vi "GetAssetList.vi"(7 "LabVIEW Web Service Request":refnum<class "Web Request.lvclass">) -> (3 "SIGMU Output":T1[](array[typedef]))   [LabVIEW 2017]
uses:
  <vilib>/wsapi/Web Request.lvclass
  typedefs/Asset Info.ctl
  typedefs/Sensor Info.ctl
  typedefs/Metric Info.ctl
  typedefs/Q_Message.ctl
panel:
  # "Use the Web Service Request input terminal to call the VIs on the Web Services palette. Do not remove it from the connector pane unless you don't need access to the palette."
  # "Each additional control wired to the connector pane will be available as an input in the URL. To include an indicator in terminal-mode output (the default setting), it must also be wired to the connector pane."
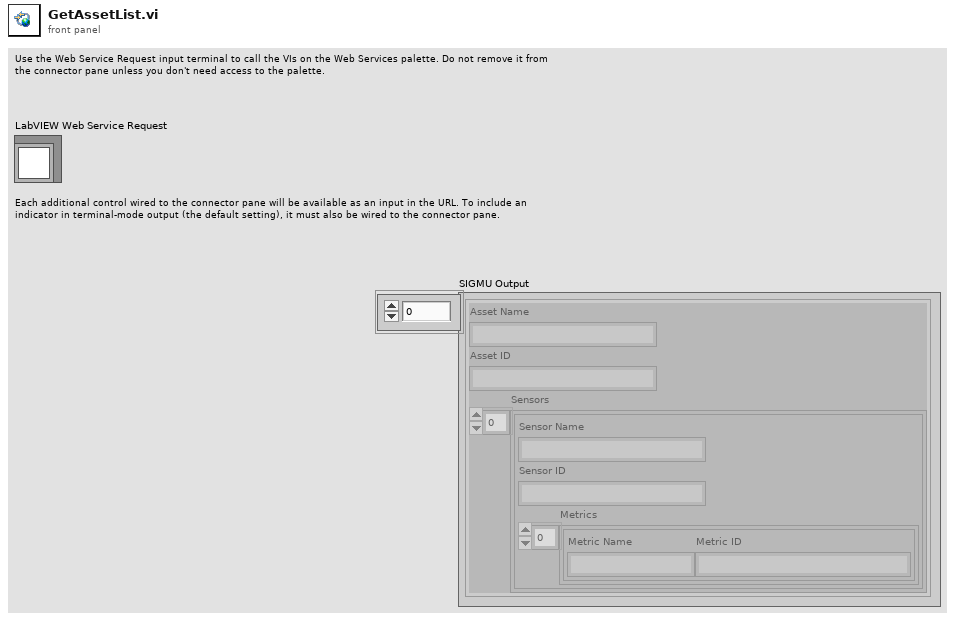
[diagram p1: front panel]
types:
  T1 = typedef "Asset Info.ctl" = cluster{"Asset Name":string, "Asset ID":string, "Sensors":T2[]}
  T2 = typedef "Sensor Info.ctl" = cluster{"Sensor Name":string, "Sensor ID":string, "Metrics":T3[]}
  T3 = typedef "Metric Info.ctl" = cluster{"Metric Name ":string, "Metric ID":string}
  T4 = typedef "Q_Message.ctl" = cluster{"Command":string, "Parameters":variant}
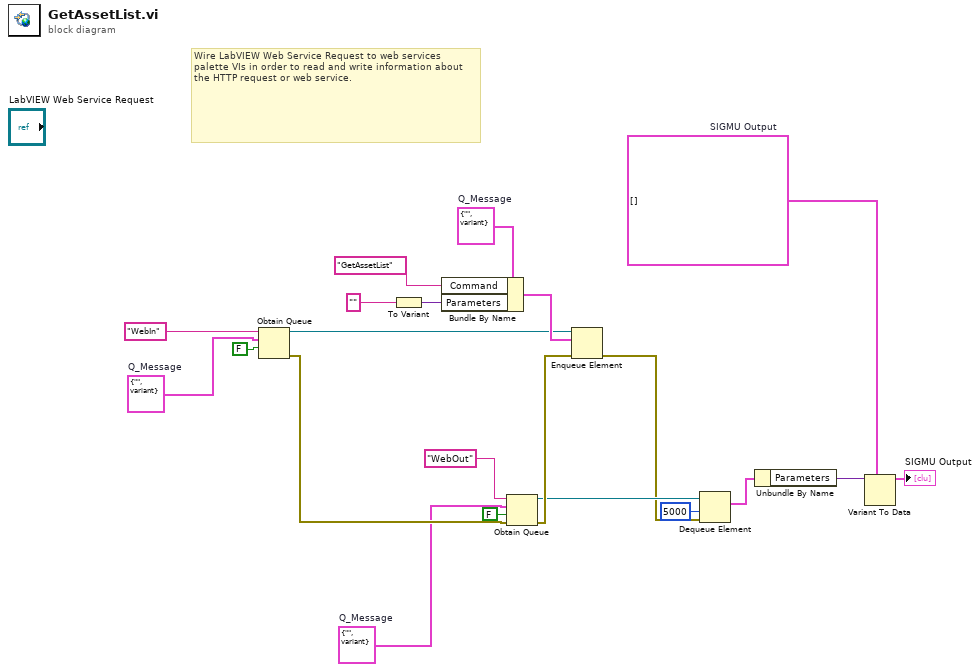
[diagram p0: block diagram]
diagram:
  w3 = T1[] []  # SIGMU Output
  w6 = T4 {"Command"="", "Parameters"=variant}  # Q_Message
  w7 = T4 {"Command"="", "Parameters"=variant}  # Q_Message
  w8 = T4 {"Command"="", "Parameters"=variant}  # Q_Message
  # "Wire LabVIEW Web Service Request to web services palette VIs in order to read and write information about the HTTP request or web service."
  n1 = Obtain Queue(name (unnamed)="WebIn", element data type=w8, create if not found? (T)=FALSE) -> (queue out=w16:refnum<queue>, error out=w14:errorcluster)  [unwired: 2 in, 1 out]
  n2 = To Variant(anything="") -> (Variant=w19:variant)
  n3 = Bundle By Name(cluster=w7, "Command"="GetAssetList", "Parameters"=w19) -> (w18:T4)
  n4 = Obtain Queue(name (unnamed)="WebOut", element data type=w6, create if not found? (T)=FALSE, error in (no error)=w14) -> (queue out=w11:refnum<queue>, error out=w12:errorcluster)  [unwired: 1 in, 1 out]
  n5 = Enqueue Element(queue=w16, element=w18, error in (no error)=w12) -> (error out=w10:errorcluster)  [unwired: 1 in, 2 out]
  n6 = Dequeue Element(queue=w11, timeout in ms (-1)=5000, error in (no error)=w10) -> (element=w5:T4)  [unwired: 3 out]
  n7 = Unbundle By Name(w5) -> ("Parameters"=w4:variant)
  n8 = Variant To Data(type=w3, Variant=w4) -> (data=→"SIGMU Output":T1[])  [unwired: 1 in, 1 out]
